vi "Get Stopped.vi"(8 "error in (no error)":errorcluster, 11 "UI_ProgressDlg in":refnum<class "UI_ProgressDlg.lvclass">) -> (0 "error out":errorcluster, 2 "Stopped?":bool, 3 "UI_ProgressDlg out":refnum<class "UI_ProgressDlg.lvclass">)   [LabVIEW 2014, in "UI_ProgressDlg.lvlib" / "UI_ProgressDlg.lvclass"]
uses:
  UI_ProgressDlg.lvclass
  UI_ProgressDlg.lvclass/UI_ProgressDlg.ctl
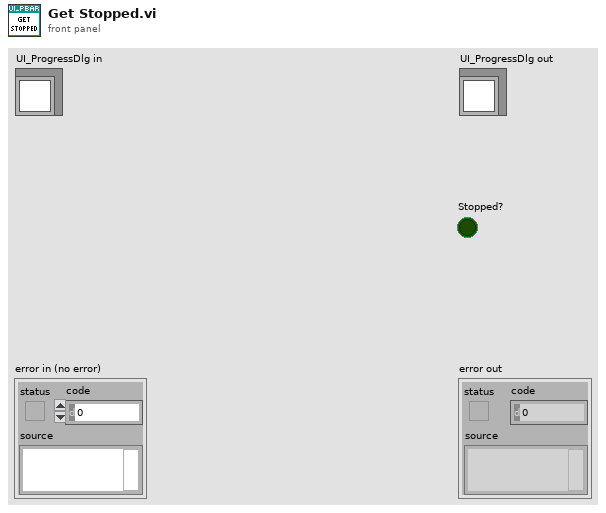
[diagram p1: front panel]
types:
  T1 = typedef "UI_ProgressDlg.lvlib/UI_ProgressDlg.lvclass/DEF-Data.ctl" = cluster{"stopped?":bool}
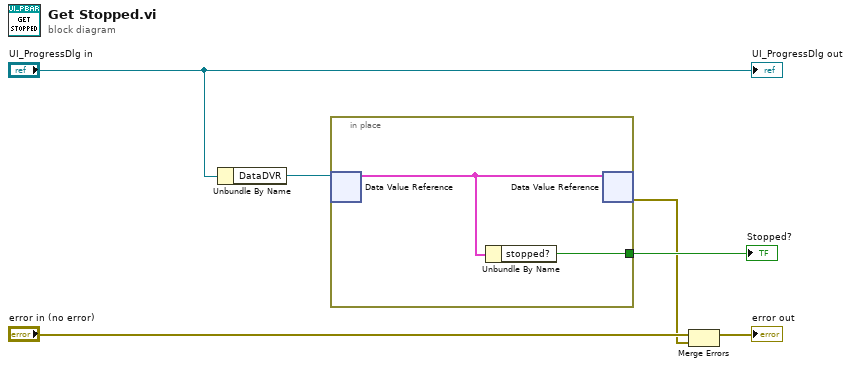
[diagram p0: block diagram]
diagram:
  n1 = Unbundle By Name("UI_ProgressDlg in") -> ("DataDVR"=w3:refnum<data-value>)
  n2 = in-place {
    in-place-border: [w7] -> w4
    n3 = in-place-dvr #1(w3) -> (w8:T1)  [unwired: 1 out]
    n4 = Unbundle By Name(w8) -> ("stopped?"=w7:bool)
    n5 = in-place-dvr #1(w8) -> (w1:errorcluster)  [unwired: 1 out]
  }
  "Stopped?" <- w4
  n6 = Merge Errors("error in (no error)", w1) -> (→"error out":errorcluster)
  "UI_ProgressDlg out" <- "UI_ProgressDlg in"
